vi "Main.vi"(11 "Module Admin":refnum<class "Delacor_lib_QMH_Cloneable Module Admin.lvclass">) -> ()   [LabVIEW 2022 SP3, in "Serial-Com-Module.lvlib"]
doc: "This template is based off of the Queued Message Handler design pattern and the Queued Message Handler project template that ships with LabVIEW.\n\nThe main difference is that the queue is private to this module and communication between modules is performed via Broadcast and Request events.\n\nRequest events are wrapped in public API methods and are handled in the Event Handling Loop (EHL) of this VI. Any module can register for Broadcast events sent by this module. The EHL generates messages based on user interface actions.\n\nThe Message Handling Loop (MHL) processes messages generated by the EHL, or by other messages. The messages are string values, so new messages can be added easily to the Message Cases case structure in the MHL. Each message cluster can also provide an optional value for Message Data, which is a variant that can be converted to whatever message-specific data is required.\n_____\nBased on DQMH Project Template 6.1.0.94."
uses:
  Serial-Com-Module.lvlib
  <vilib>/Delacor/Delacor QMH/Libraries/Message Queue_class/Delacor_lib_QMH_Message Queue.lvclass
  Module Data--cluster.ctl
  <vilib>/Utility/miscctls.llb/LVPointTypeDef.ctl
  <vilib>/Utility/error.llb/Error Cluster From Error Code.vi
  <vilib>/ErrorRing/Error Ring.xnode
  <vilib>/Delacor/Delacor QMH/Libraries/Message Queue_class/Delacor_lib_QMH_Enqueue Message (Single).vi
  Stop Argument--cluster.ctl
  <vilib>/Delacor/Delacor QMH/Libraries/Cloneable Module Admin_class/Delacor_lib_QMH_Cloneable Module Admin.lvclass
  Dependencies/Serial-Com-Library.lvlibp/Serial Base Class/Serial Base.lvclass
  Init Serial (Reply Payload)--cluster.ctl
  Dependencies/Serial-Com-Library.lvlibp/Serial Base Class/Object Argument--cluster.ctl
  Init Serial Argument--cluster.ctl
  Open Port (Reply Payload)--cluster.ctl
  Open Port Argument--cluster.ctl
  Close Port (Reply Payload)--cluster.ctl
  Close Port Argument--cluster.ctl
  Read Buffer (Reply Payload)--cluster.ctl
  Read Buffer Argument--cluster.ctl
  Send (Reply Payload)--cluster.ctl
  Send Argument--cluster.ctl
  Send Line (Reply Payload)--cluster.ctl
  Dependencies/Serial-Com-Library.lvlibp/Serial Base Class/Termination Character--enum.ctl
  Send Line Argument--cluster.ctl
panel:
  out "error out":errorcluster
  out "Status":string
  in  "Simulate EHL Error":bool
  in  "Simulate MHL Error":bool
  # "Other QMH Modules communicate with this Module via its Public API (wrappers for its Request Events).\n\nThis Module communicates with other Modules via its Broadcast Events.\nAny module that wants to get these messages, just registers for this module's Broadcast events."
  # "This template is for the Delacor Modified Queued Message Handler design pattern.\n\nSee the block diagram for more information on how to use this template."
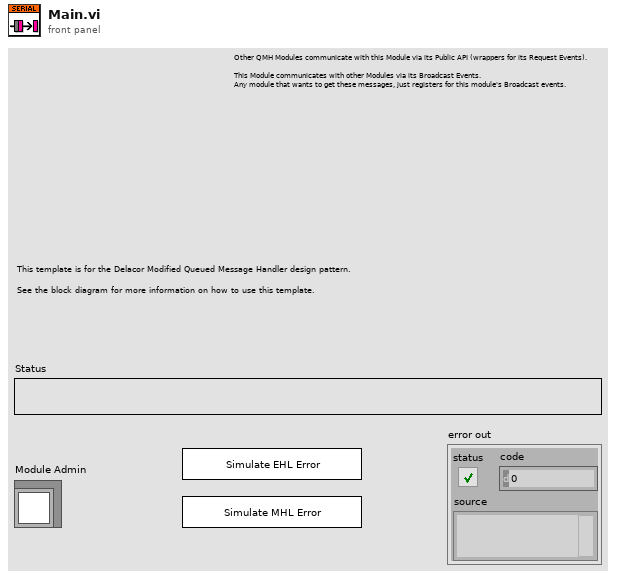
[diagram p1: front panel]
types:
  T1 = typedef "Serial-Com-Module.lvlib/Request Events--cluster.ctl" = cluster{"Stop Module":refnum<user-event>, "Show Panel":refnum<user-event>, "Hide Panel":refnum<user-event>, "Show Diagram":refnum<user-event>, "Get Module Execution Status":refnum<user-event>, "Init Serial":refnum<user-event>, "Open Port":refnum<user-event>, "Close Port":refnum<user-event>, "Read Buffer":refnum<user-event>, "Send":refnum<user-event>, "Send Line":refnum<user-event>}
  T2 = typedef "Serial-Com-Module.lvlib/Module Data--cluster.ctl" = cluster{"Status":string, "Serial Com Obj":refnum<class "Serial Base.lvclass">}
  T3 = enum32{"invalid lock state", "Not Locked", "Locked (No Password)", "Password-protected"}
  T4 = typedef "Serial-Com-Module.lvlib/Stop Argument--cluster.ctl" = cluster{"Module ID":i32, "Origin":string, "Exit via Stop Module Req?":bool, "Wait for Module to stop?":bool}
  T5 = typedef "Serial-Com-Module.lvlib/Init Serial Argument--cluster.ctl" = cluster{"Module ID":i32, "Serial Config":T6, "Wait Notifier":refnum<notifier>, "wait for reply":bool}
  T6 = typedef "Serial-Com-Library.lvlibp/Serial Base.lvclass/Object Argument--cluster.ctl" = cluster{"Com Port":refnum<visa-resource-name>, "baud rate":u32, "data bits":u16, "parity":enum16{"None", "Odd", "Even", "Mark", "Space"}, "timeout ":u32}
  T7 = typedef "Serial-Com-Module.lvlib/Open Port Argument--cluster.ctl" = cluster{"Module ID":i32, "Open Port?":bool, "Wait Notifier":refnum<notifier>, "wait for reply":bool}
  T8 = typedef "Serial-Com-Module.lvlib/Close Port Argument--cluster.ctl" = cluster{"Module ID":i32, "ClosePort?":bool, "Wait Notifier":refnum<notifier>, "wait for reply":bool}
  T9 = typedef "Serial-Com-Module.lvlib/Read Buffer Argument--cluster.ctl" = cluster{"Module ID":i32, "pre-read delay":i16, "Wait Notifier":refnum<notifier>, "wait for reply":bool}
  T10 = typedef "Serial-Com-Module.lvlib/Send Argument--cluster.ctl" = cluster{"Module ID":i32, "data":string, "Wait Notifier":refnum<notifier>, "wait for reply":bool}
  T11 = typedef "Serial-Com-Module.lvlib/Send Line Argument--cluster.ctl" = cluster{"Module ID":i32, "Termination Char":T12, "data":string, "Wait Notifier":refnum<notifier>, "wait for reply":bool}
  T12 = typedef "Serial-Com-Library.lvlibp/Serial Base.lvclass/Termination Character--enum.ctl" = enum16{"none", "\\r\\n", "\\r", "\\n"}
  T13 = typedef "LVPointTypeDef.ctl" = cluster{"Horizontal":i16, "Vertical":i16}
  T14 = enum32{"Invalid", "Standard", "Closed", "Hidden", "Minimized", "Maximized"}
  T15 = typedef "Serial-Com-Module.lvlib/Init Serial (Reply Payload)--cluster.ctl" = cluster{"error":errorcluster}
  T16 = typedef "Serial-Com-Module.lvlib/Open Port (Reply Payload)--cluster.ctl" = cluster{"error":errorcluster}
  T17 = typedef "Serial-Com-Module.lvlib/Close Port (Reply Payload)--cluster.ctl" = cluster{"error":errorcluster}
  T18 = typedef "Serial-Com-Module.lvlib/Read Buffer (Reply Payload)--cluster.ctl" = cluster{"buffer output":string, "bytes count":i16, "error":errorcluster}
  T19 = typedef "Serial-Com-Module.lvlib/Send (Reply Payload)--cluster.ctl" = cluster{"bytes count sent":u32, "error":errorcluster}
  T20 = typedef "Serial-Com-Module.lvlib/Send Line (Reply Payload)--cluster.ctl" = cluster{"bytes count":u32, "error":errorcluster}
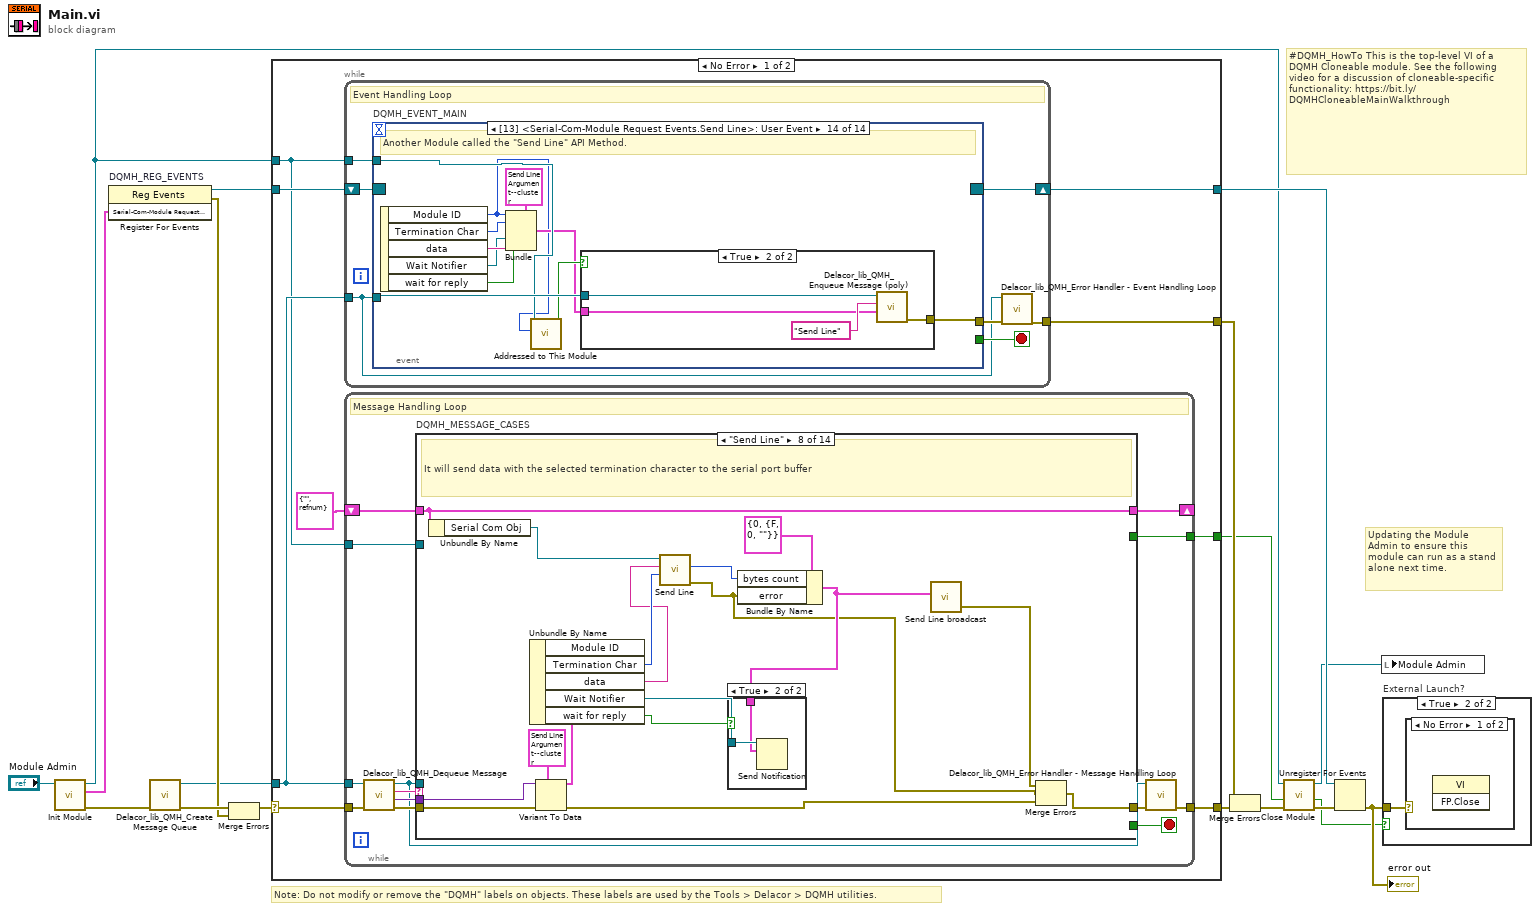
[diagram p0: block diagram]
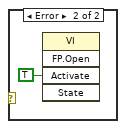
[diagram p3: hidden frame]
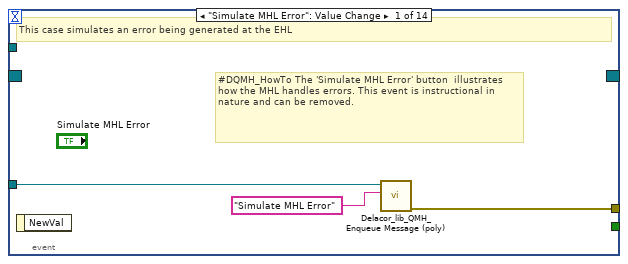
[diagram p4: hidden frame]
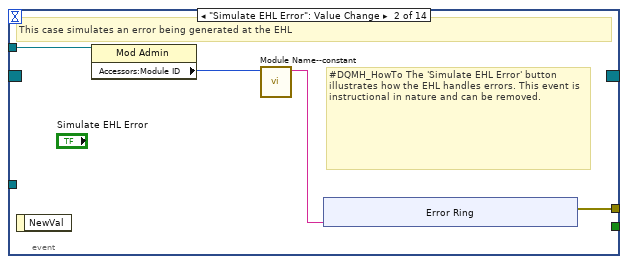
[diagram p5: hidden frame]
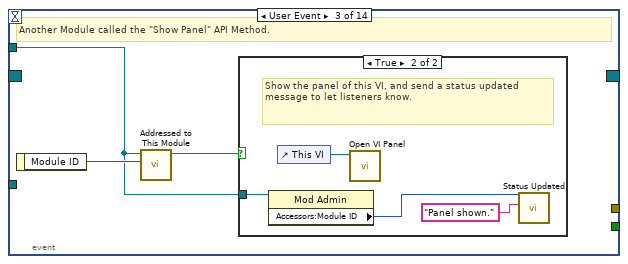
[diagram p6: hidden frame]
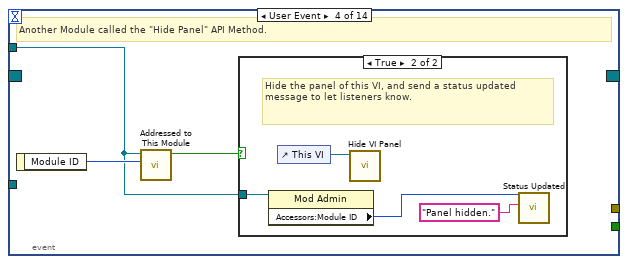
[diagram p8: hidden frame]
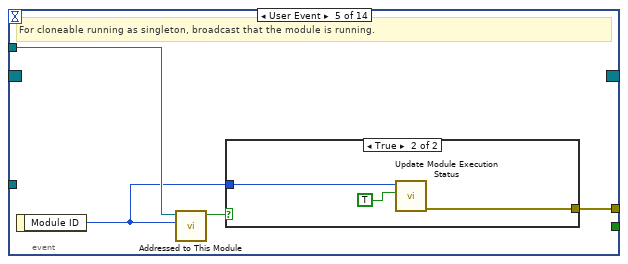
[diagram p10: hidden frame]
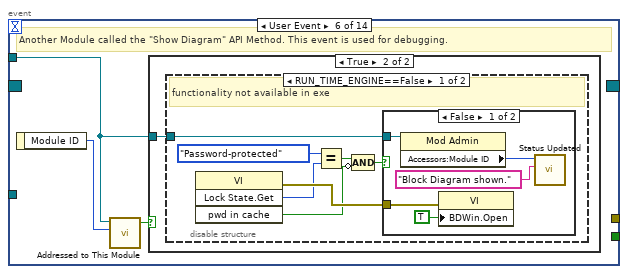
[diagram p12: hidden frame]
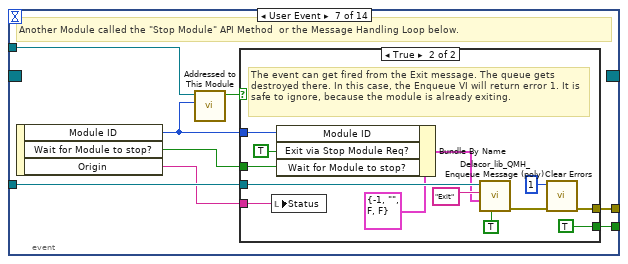
[diagram p16: hidden frame]
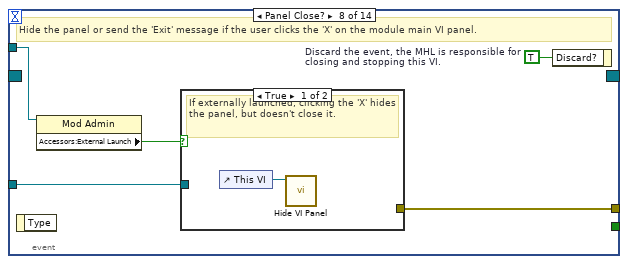
[diagram p18: hidden frame]
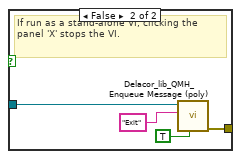
[diagram p19: hidden frame]
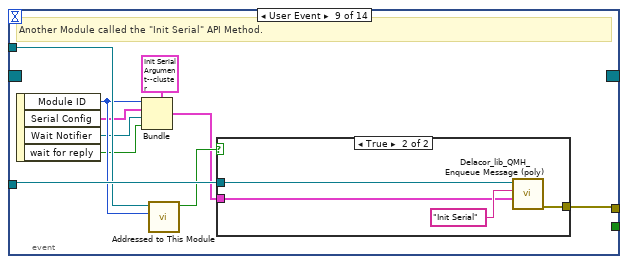
[diagram p20: hidden frame]
diagram:
  # "#DQMH_HowTo This is the top-level VI of a DQMH Cloneable module. See the following video for a discussion of cloneable-specific functionality: https://bit.ly/DQMHCloneableMainWalkthrough"
  # "Note: Do not modify or remove the \"DQMH\" labels on objects. These labels are used by the Tools > Delacor > DQMH utilities."
  # "Updating the Module Admin to ensure this module can run as a stand alone next time."
  n1 = call "Init Module.vi"("Cloneable Module Admin in"="Module Admin") -> ("error out"=w15:errorcluster, "Serial-Com-Module Request Events"=w7:T1, "Cloneable Module Admin out"=w4:refnum<class "Delacor_lib_QMH_Cloneable Module Admin.lvclass">)  [unwired: 8 in]
  n2 = register-events "DQMH_REG_EVENTS"(w7) -> (reference out=w8:refnum<event-registration>, error out=w10:errorcluster)  [unwired: 2 in]
  n3 = call <vilib>:"Delacor_lib_QMH_Create Message Queue.vi"("error in"=w15) -> ("error out"=w12:errorcluster, "Message Queue"=w6:refnum<class "Delacor_lib_QMH_Message Queue.lvclass">)  [unwired: 9 in]
  n4 = Merge Errors(w12, w10) -> (w11:errorcluster)
  n5 = case shown="No Error" w11 {
    selector: w11 -> [w25 w428]
    tunnel: [w27 w427] -> w16
    tunnel: [w24 w435] -> w9
    tunnel: w8 -> [w22 w435]
    tunnel: w6 -> [w21 w426]
    tunnel: [w26 _] -> w17
    tunnel: w4 -> [w20 w431]
    tunnel: [w19 _] -> w2
    frame No Error {
      n6 = while {
        tunnel: w21 -> [w28]
        shift-right: [w31] -> w24
        shift-left: w22 -> [w32]
        tunnel: [w33] -> w26
        tunnel: w20 -> [w29]
        stop <- w30 stop-if-true
        # "Event Handling Loop"
        n7 = event "DQMH_EVENT_MAIN" shown="[13] <Serial-Com-Module Request Events.Send Line>: User Event" {
          selector: w32 -> [_ _ _ _ _ _ _ _ _ _ _ _ _ _]
          dyn-events: [_ _ _ _ _ _ _ _ _ _ _ _ _ _] -> w31
          timeout: _ -> [_ _ _ _ _ _ _ _ _ _ _ _ _ _]
          tunnel: [_ _ _ _ _ _ w89 _ _ _ _ _ _ _] -> w30
          tunnel: w28 -> [w36 _ _ _ _ _ w92 w108 w126 w140 w154 w168 w182 w197]
          tunnel: [w37 w41 _ _ w66 _ w93 w111 w117 w131 w145 w159 w173 w187] -> w34
          tunnel: w29 -> [_ w40 w49 w56 w64 w70 w91 w109 w124 w138 w152 w166 w180 w195]
          event "Simulate MHL Error": Value Change {
            # "#DQMH_HowTo The 'Simulate MHL Error' button  illustrates how the MHL handles errors. This event is instructional in nature and can be removed."
            # "This case simulates an error being generated at the EHL"
            n8 = event-data() -> ()  [unwired: 1 in, 1 out]
            n9 = call-poly <vilib>:"Delacor_lib_QMH_Enqueue Message (poly).vi"("Message"="Simulate MHL Error", "Message Queue in"=w36) -> ("error out"=w37:errorcluster)  [unwired: 8 in, 1 out]
          }
          event "Simulate EHL Error": Value Change {
            # "#DQMH_HowTo The 'Simulate EHL Error' button  illustrates how the EHL handles errors. This event is instructional in nature and can be removed."
            # "This case simulates an error being generated at the EHL"
            n10 = event-data() -> ()  [unwired: 1 in, 1 out]
            n11 = property class="Mod Admin"(reference=w40) -> ("Accessors:Module ID"=w39:i32)  [unwired: 1 in, 2 out]
            n12 = call "Module Name--constant.vi"("Module ID"=w39) -> ("Module Name"=w38:string)  [unwired: 10 in]
            n13 = xnode "Error Ring"("parameter 0"=w38) -> ("error out"=w41:errorcluster)
          }
          event User Event {
            # "Another Module called the \"Show Panel\" API Method."
            n14 = event-data() -> ("Module ID"=w50:i32)  [unwired: 1 in]
            n15 = call "Addressed to This Module.vi"("Module ID from Argument"=w50, "Module Admin"=w49) -> ("Addressed to this instance?"=w51:bool)  [unwired: 8 in, 1 out]
            n16 = case shown="True" w51 {
              tunnel: w49 -> [_ w53]
              frame False {
              }
              frame True {
                # "Show the panel of this VI, and send a status updated message to let listeners know."
                n17 = property class="Mod Admin"(reference=w53) -> ("Accessors:Module ID"=w52:i32)  [unwired: 1 in, 2 out]
                n18 = control-ref of="This VI"() -> (w55:refnum<vi>)
                n19 = call "Open VI Panel.vi"("VI"=w55) -> ()  [unwired: 10 in, 1 out]
                n20 = call "Status Updated.vi"("Status"="Panel shown." ("format string"), "Module ID"=w52) -> ()  [unwired: 9 in, 1 out]
              }
            }
          }
          event User Event {
            # "Another Module called the \"Hide Panel\" API Method."
            n21 = event-data() -> ("Module ID"=w57:i32)  [unwired: 1 in]
            n22 = call "Addressed to This Module.vi"("Module ID from Argument"=w57, "Module Admin"=w56) -> ("Addressed to this instance?"=w58:bool)  [unwired: 8 in, 1 out]
            n23 = case shown="True" w58 {
              tunnel: w56 -> [_ w60]
              frame False {
              }
              frame True {
                # "Hide the panel of this VI, and send a status updated message to let listeners know."
                n24 = property class="Mod Admin"(reference=w60) -> ("Accessors:Module ID"=w59:i32)  [unwired: 1 in, 2 out]
                n25 = control-ref of="This VI"() -> (w62:refnum<vi>)
                n26 = call "Hide VI Panel.vi"("VI"=w62) -> ()  [unwired: 10 in, 1 out]
                n27 = call "Status Updated.vi"("Status"="Panel hidden." ("format string"), "Module ID"=w59) -> ()  [unwired: 9 in, 1 out]
              }
            }
          }
          event User Event {
            # "For cloneable running as singleton, broadcast that the module is running."
            n28 = event-data() -> ("Module ID"=w63:i32)  [unwired: 1 in]
            n29 = call "Addressed to This Module.vi"("Module ID from Argument"=w63, "Module Admin"=w64) -> ("Addressed to this instance?"=w65:bool)  [unwired: 8 in, 1 out]
            n30 = case shown="True" w65 {
              tunnel: [_ w69] -> w66
              tunnel: w63 -> [_ w68]
              frame False {
              }
              frame True {
                n31 = call "Update Module Execution Status.vi"("Running?"=TRUE, "Module ID"=w68) -> ("error out"=w69:errorcluster)  [unwired: 9 in]
              }
            }
          }
          event User Event {
            # "Another Module called the \"Show Diagram\" API Method. This event is used for debugging."
            n32 = event-data() -> ("Module ID"=w71:i32)  [unwired: 1 in]
            n33 = call "Addressed to This Module.vi"("Module ID from Argument"=w71, "Module Admin"=w70) -> ("Addressed to this instance?"=w72:bool)  [unwired: 8 in, 1 out]
            n34 = case shown="True" w72 {
              tunnel: w70 -> [_ w73]
              frame False {
              }
              frame True {
                n35 = disable-structure shown="RUN_TIME_ENGINE==False" {
                  disable-tunnel: w73 -> [w74 _]
                  frame condition #0 (active) {
                    # "functionality not available in exe"
                    n36 = invoke class="VI" method="Lock State.Get"() -> (error out=w80:errorcluster, "Get Lock State"=w79:T3, "pwd in cache"=w76:bool)  [unwired: 4 in, 1 out]
                    n37 = Equal?(x=T3."Password-protected", y=w79) -> (x = y?=w77:bool)
                    n38 = Compound Arithmetic op=AND(w77, invert w76) -> (w75:bool)
                    n39 = case shown="False" w75 {
                      tunnel: w80 -> [w85 _]
                      tunnel: w74 -> [w82 _]
                      frame False {
                        n40 = property class="Mod Admin"(reference=w82) -> ("Accessors:Module ID"=w81:i32)  [unwired: 1 in, 2 out]
                        n41 = property class="VI"(error in=w85, "BDWin.Open"=TRUE ("Block Diagram Window:Open")) -> ()  [unwired: 1 in, 2 out]
                        n42 = call "Status Updated.vi"("Status"="Block Diagram shown." ("format string"), "Module ID"=w81) -> ()  [unwired: 9 in, 1 out]
                      }
                      frame True {
                        # "Password-protected VI, and the password is not in the cache. Do not show the diagram."
                      }
                    }
                  }
                  frame condition #1 {
                  }
                }
              }
            }
          }
          event User Event {
            # "Another Module called the \"Stop Module\" API Method  or the Message Handling Loop below."
            n43 = event-data() -> ("Module ID"=w87:i32, "Wait for Module to stop?"=w88:bool, "Origin"=w86:string)  [unwired: 1 in]
            n44 = call "Addressed to This Module.vi"("Module ID from Argument"=w87, "Module Admin"=w91) -> ("Addressed to this instance?"=w90:bool)  [unwired: 8 in, 1 out]
            n45 = case shown="True" w90 {
              tunnel: [_ w105] -> w93
              tunnel: w92 -> [_ w101]
              tunnel: [_ TRUE] -> w89
              tunnel: w88 -> [_ w96]
              tunnel: w87 -> [_ w98]
              tunnel: w86 -> [_ w94]
              frame False {
              }
              frame True {
                # "The event can get fired from the Exit message. The queue gets destroyed there. In this case, the Enqueue VI will return error 1. It is safe to ignore, because the module is already exiting."
                n46 = local write "Status"(w94) -> ()
                n47 = Bundle By Name(cluster=T4 {"Module ID"=-1, "Origin"="", "Exit via Stop Module Req?"=FALSE, "Wait for Module to stop?"=FALSE} ("Stop Argument"), "Module ID"=w98, "Exit via Stop Module Req?"=TRUE, "Wait for Module to stop?"=w96) -> (w95:T4)
                n48 = call-poly <vilib>:"Delacor_lib_QMH_Enqueue Message (poly).vi"("Priority Message? (F)"=TRUE, "Message Data"=w95, "Message"="Exit", "Message Queue in"=w101) -> ("error out"=w106:errorcluster)  [unwired: 6 in, 1 out]
                n49 = call <vilib>:"Clear Errors.vi"("error in (no error)"=w106, "specific error code to clear (0: all)"=1) -> ("error out"=w105:errorcluster)  [unwired: 4 in, 1 out]
              }
            }
          }
          event Panel Close? {
            w110 = TRUE  # Discard the event, the MHL is responsible for closing and stopping this VI.
            # "Hide the panel or send the 'Exit' message if the user clicks the 'X' on the module main VI panel."
            n50 = event-data() -> ()  [unwired: 1 in, 1 out]
            n51 = property class="Mod Admin"(reference=w109) -> ("Accessors:External Launch"=w107:bool)  [unwired: 1 in, 2 out]
            n52 = case shown="True" w107 {
              tunnel: w108 -> [_ w115]
              tunnel: [_ w116] -> w111
              frame True {
                # "If externally launched, clicking the 'X' hides the panel, but doesn't close it."
                n53 = control-ref of="This VI"() -> (w112:refnum<vi>)
                n54 = call "Hide VI Panel.vi"("VI"=w112) -> ()  [unwired: 10 in, 1 out]
              }
              frame False {
                # "If run as a stand-alone VI, clicking the panel 'X' stops the VI."
                n55 = call-poly <vilib>:"Delacor_lib_QMH_Enqueue Message (poly).vi"("Priority Message? (F)"=TRUE, "Message"="Exit", "Message Queue in"=w115) -> ("error out"=w116:errorcluster)  [unwired: 7 in, 1 out]
              }
            }
            n56 = event-data("Discard?"=w110) -> ()  [unwired: 1 in, 1 out]
          }
          event User Event {
            # "Another Module called the \"Init Serial\" API Method."
            n57 = event-data() -> ("Module ID"=w121:i32, "Serial Config"=w120:T6, "Wait Notifier"=w119:refnum<notifier>, "wait for reply"=w118:bool)  [unwired: 1 in]
            n58 = Bundle(cluster=T5 {"Module ID"=-1, "Serial Config"={"Com Port"="", "baud rate"=0, "data bits"=8, "parity"=enum."None", "timeout "=10000}, "Wait Notifier"=refnum, "wait for reply"=FALSE} ("Init Serial Argument"), "Module ID"=w121, "Serial Config"=w120, "Wait Notifier"=w119, "wait for reply"=w118) -> (w122:T5)
            n59 = call "Addressed to This Module.vi"("Module ID from Argument"=w121, "Module Admin"=w124) -> ("Addressed to this instance?"=w125:bool)  [unwired: 8 in, 1 out]
            n60 = case shown="True" w125 {
              tunnel: w126 -> [_ w130]
              tunnel: w122 -> [_ w128]
              tunnel: [_ w127] -> w117
              frame False {
              }
              frame True {
                n61 = call-poly <vilib>:"Delacor_lib_QMH_Enqueue Message (poly).vi"("Message Data"=w128, "Message"="Init Serial", "Message Queue in"=w130) -> ("error out"=w127:errorcluster)  [unwired: 7 in, 1 out]
              }
            }
          }
          event User Event {
            # "Another Module called the \"Open Port\" API Method."
            n62 = event-data() -> ("Module ID"=w135:i32, "Open Port?"=w134:bool, "Wait Notifier"=w133:refnum<notifier>, "wait for reply"=w132:bool)  [unwired: 1 in]
            n63 = Bundle(cluster=T7 {"Module ID"=-1, "Open Port?"=FALSE, "Wait Notifier"=refnum, "wait for reply"=FALSE} ("Open Port Argument"), "Module ID"=w135, "Open Port?"=w134, "Wait Notifier"=w133, "wait for reply"=w132) -> (w136:T7)
            n64 = call "Addressed to This Module.vi"("Module ID from Argument"=w135, "Module Admin"=w138) -> ("Addressed to this instance?"=w139:bool)  [unwired: 8 in, 1 out]
            n65 = case shown="True" w139 {
              tunnel: w140 -> [_ w144]
              tunnel: w136 -> [_ w142]
              tunnel: [_ w141] -> w131
              frame False {
              }
              frame True {
                n66 = call-poly <vilib>:"Delacor_lib_QMH_Enqueue Message (poly).vi"("Message Data"=w142, "Message"="Open Port", "Message Queue in"=w144) -> ("error out"=w141:errorcluster)  [unwired: 7 in, 1 out]
              }
            }
          }
          event User Event {
            # "Another Module called the \"Close Port\" API Method."
            n67 = event-data() -> ("Module ID"=w149:i32, "ClosePort?"=w148:bool, "Wait Notifier"=w147:refnum<notifier>, "wait for reply"=w146:bool)  [unwired: 1 in]
            n68 = Bundle(cluster=T8 {"Module ID"=-1, "ClosePort?"=FALSE, "Wait Notifier"=refnum, "wait for reply"=FALSE} ("Close Port Argument"), "Module ID"=w149, "ClosePort?"=w148, "Wait Notifier"=w147, "wait for reply"=w146) -> (w150:T8)
            n69 = call "Addressed to This Module.vi"("Module ID from Argument"=w149, "Module Admin"=w152) -> ("Addressed to this instance?"=w153:bool)  [unwired: 8 in, 1 out]
            n70 = case shown="True" w153 {
              tunnel: w154 -> [_ w158]
              tunnel: w150 -> [_ w156]
              tunnel: [_ w155] -> w145
              frame False {
              }
              frame True {
                n71 = call-poly <vilib>:"Delacor_lib_QMH_Enqueue Message (poly).vi"("Message Data"=w156, "Message"="Close Port", "Message Queue in"=w158) -> ("error out"=w155:errorcluster)  [unwired: 7 in, 1 out]
              }
            }
          }
          event User Event {
            # "Another Module called the \"Read Buffer\" API Method."
            n72 = event-data() -> ("Module ID"=w163:i32, "pre-read delay"=w162:i16, "Wait Notifier"=w161:refnum<notifier>, "wait for reply"=w160:bool)  [unwired: 1 in]
            n73 = Bundle(cluster=T9 {"Module ID"=-1, "pre-read delay"=-1, "Wait Notifier"=refnum, "wait for reply"=FALSE} ("Read Buffer Argument"), "Module ID"=w163, "pre-read delay"=w162, "Wait Notifier"=w161, "wait for reply"=w160) -> (w164:T9)
            n74 = call "Addressed to This Module.vi"("Module ID from Argument"=w163, "Module Admin"=w166) -> ("Addressed to this instance?"=w167:bool)  [unwired: 8 in, 1 out]
            n75 = case shown="True" w167 {
              tunnel: w168 -> [_ w172]
              tunnel: w164 -> [_ w170]
              tunnel: [_ w169] -> w159
              frame False {
              }
              frame True {
                n76 = call-poly <vilib>:"Delacor_lib_QMH_Enqueue Message (poly).vi"("Message Data"=w170, "Message"="Read Buffer", "Message Queue in"=w172) -> ("error out"=w169:errorcluster)  [unwired: 7 in, 1 out]
              }
            }
          }
          event User Event {
            # "Another Module called the \"Send\" API Method."
            n77 = event-data() -> ("Module ID"=w177:i32, "data"=w176:string, "Wait Notifier"=w175:refnum<notifier>, "wait for reply"=w174:bool)  [unwired: 1 in]
            n78 = Bundle(cluster=T10 {"Module ID"=-1, "data"="", "Wait Notifier"=refnum, "wait for reply"=FALSE} ("Send Argument"), "Module ID"=w177, "data"=w176, "Wait Notifier"=w175, "wait for reply"=w174) -> (w178:T10)
            n79 = call "Addressed to This Module.vi"("Module ID from Argument"=w177, "Module Admin"=w180) -> ("Addressed to this instance?"=w181:bool)  [unwired: 8 in, 1 out]
            n80 = case shown="True" w181 {
              tunnel: w182 -> [_ w186]
              tunnel: w178 -> [_ w184]
              tunnel: [_ w183] -> w173
              frame False {
              }
              frame True {
                n81 = call-poly <vilib>:"Delacor_lib_QMH_Enqueue Message (poly).vi"("Message Data"=w184, "Message"="Send", "Message Queue in"=w186) -> ("error out"=w183:errorcluster)  [unwired: 7 in, 1 out]
              }
            }
          }
          event User Event {
            # "Another Module called the \"Send Line\" API Method."
            n82 = event-data() -> ("Module ID"=w192:i32, "Termination Char"=w191:T12, "data"=w190:string, "Wait Notifier"=w189:refnum<notifier>, "wait for reply"=w188:bool)  [unwired: 1 in]
            n83 = Bundle(cluster=T11 {"Module ID"=-1, "Termination Char"=enum."none", "data"="", "Wait Notifier"=refnum, "wait for reply"=FALSE} ("Send Line Argument"), "Module ID"=w192, "Termination Char"=w191, "data"=w190, "Wait Notifier"=w189, "wait for reply"=w188) -> (w193:T11)
            n84 = call "Addressed to This Module.vi"("Module ID from Argument"=w192, "Module Admin"=w195) -> ("Addressed to this instance?"=w196:bool)  [unwired: 8 in, 1 out]
            n85 = case shown="True" w196 {
              tunnel: w197 -> [_ w201]
              tunnel: w193 -> [_ w199]
              tunnel: [_ w198] -> w187
              frame False {
              }
              frame True {
                n86 = call-poly <vilib>:"Delacor_lib_QMH_Enqueue Message (poly).vi"("Message Data"=w199, "Message"="Send Line", "Message Queue in"=w201) -> ("error out"=w198:errorcluster)  [unwired: 7 in, 1 out]
              }
            }
          }
        }
        n87 = call-dynamic "Delacor_lib_QMH_Error Handler - Event Handling Loop.vi"("error in"=w34, "Message Queue in"=w28) -> ("dup error in"=w33:errorcluster)  [unwired: 8 in, 1 out]
      }
      n88 = while {
        tunnel: w21 -> [w205]
        shift-right: [w209] -> _
        shift-left: T2 {"Status"="", "Serial Com Obj"=refnum} ("Data Cluster") -> [w210]
        tunnel: w25 -> [w213]
        tunnel: [w211] -> w27
        tunnel: w20 -> [w203]
        tunnel: [w202] -> w19
        stop <- w208 stop-if-true
        # "Message Handling Loop"
        n89 = call-dynamic "Delacor_lib_QMH_Dequeue Message.vi"("error in"=w213, "Message Queue in"=w205) -> ("error out"=w212:errorcluster, "Message Data"=w206:variant, "Message"=w207:string, "Message Queue out"=w204:refnum<class "Delacor_lib_QMH_Message Queue.lvclass">)  [unwired: 6 in]
        n90 = case "DQMH_MESSAGE_CASES" shown="\"Send Line\"" w207 {
          selector: w207 -> [_ _ _ _ _ _ _ _ _ _ _ _ _ w413]
          tunnel: w204 -> [_ _ _ _ _ _ _ _ _ _ w364 _ w403 _]
          tunnel: w212 -> [w233 w237 w250 w277 w295 w316 w336 w355 w360 w362 w373 w386 w409 w415]
          tunnel: [w231 w237 w244 w270 w286 w307 w327 w346 w359 w362 w369 w385 w406 w416] -> w214
          tunnel: w210 -> [w224 w236 w243 w268 w284 w302 w323 w345 w358 w361 w368 w383 w402 w414]
          tunnel: [w223 w236 w242 w267 w282 w300 w322 w345 w358 w361 w368 w383 w402 w414] -> w209
          tunnel: [_ _ _ _ _ _ _ _ _ _ _ _ w401 _] -> w208
          tunnel: w206 -> [_ _ w249 w275 w293 w314 w334 w353 _ _ w367 _ w399 _]
          tunnel: w203 -> [w218 _ _ _ _ _ _ _ _ _ w366 w381 w395 w411]
          tunnel: [_ _ _ _ _ _ _ _ _ _ _ _ w397 _] -> w202
          frame "Initialize" {
            w215 = "Initial Message" ("Initial Message")
            # "#CodeNeeded - Initialize the appearance of the front panel."
            # "#CodeNeeded - Initialize your state data here."
            # "Initialize - Any operation that needs to be done before the module can receive messages. Synchronize Caller Events.vi will inform Start Module.vi that the module has launched and is ready to receive messages. Module Did Init.vi will broadcast that the module initialized."
            n91 = call "Synchronize Caller Events.vi"("error in (no error)"=w233, "Module Admin"=w218) -> ("error out"=w232:errorcluster, "Module Admin out"=w217:refnum<class "Delacor_lib_QMH_Cloneable Module Admin.lvclass">)  [unwired: 8 in]
            n92 = property class="Mod Admin"(reference=w217) -> ("Accessors:Module ID"=w220:i32, "Accessors:External Launch"=w219:bool)  [unwired: 1 in, 2 out]
            n93 = call "Module Name--constant.vi"("Module ID"=w220) -> ("Module Name"=w228:string)  [unwired: 10 in]
            n94 = property class="VI"("Front Panel.Title"=w228) -> (reference out=w230:refnum<vi>, error out=w235:errorcluster)  [unwired: 2 in]
            n95 = Select(t=T14."Hidden" ("State"), s=w219, f=T14."Standard" ("State")) -> (s? t:f=w225:T14)
            n96 = invoke class="VI" method="FP.Open"(reference=w230, error in=w235, "State"=w225) -> (reference out=w229:refnum<vi>, error out=w234:errorcluster)  [unwired: 2 in, 3 out]
            n97 = call "Module Name--constant.vi"("Module ID"=w220) -> ("Module Name"=w221:string)  [unwired: 10 in]
            n98 = Bundle By Name(cluster=w224, "Status"=w215) -> (w223:T2)
            n99 = invoke class="VI" method="FP.Center"(reference=w229, error in=w234) -> ()  [unwired: 1 in, 3 out]
            n100 = property on="Pane" class="Pane"("Origin"=T13 {"Horizontal"=0, "Vertical"=0}) -> ()  [unwired: 2 in, 2 out]
            n101 = call "Module Did Init.vi"("error in (no error)"=w232, "Initialized?"=TRUE, "Origin"=w221, "Module ID"=w220) -> ("error out"=w231:errorcluster)  [unwired: 7 in]
            "Status" <- w215
          }
          frame "---Module Specific---" {
            # "Separator -- The following cases handle messages specific to this Module."
          }
          frame "Init Serial" {
            # "It will populate the config parameters required before open the serial port"
            n102 = Variant To Data(error in=w250, type=T5 {"Module ID"=-1, "Serial Config"={"Com Port"="", "baud rate"=0, "data bits"=8, "parity"=enum."None", "timeout "=10000}, "Wait Notifier"=refnum, "wait for reply"=FALSE} ("Init Serial Argument"), Variant=w249) -> (data=w247:T5, error out=w241:errorcluster)
            n103 = Unbundle By Name(w247) -> ("Serial Config"=w239:T6, "Wait Notifier"=w246:refnum<notifier>, "wait for reply"=w245:bool)  [unwired: 1 out]
            n104 = case shown="True" w245 {
              tunnel: w246 -> [_ w261]
              tunnel: w239 -> [_ w258]
              tunnel: [errorcluster {"status"=FALSE, "code"=0, "source"=""} ("error out") w256] -> w240
              tunnel: [refnum<class "Serial Base.lvclass"> refnum ("Serial-Com-Library.lvlibp:Serial Base.lvclass") w255] -> w238
              frame False {
              }
              frame True {
                n105 = call-dynamic "Init.vi"("error in (no error)"=errorcluster {"status"=FALSE, "code"=0, "source"=""}, "Serial Config"=w258, "Serial Base in"=refnum<class "Serial Base.lvclass"> refnum ("Serial-Com-Library.lvlibp:Serial Base.lvclass")) -> ("error out"=w254:errorcluster, "Serial Base out"=w255:refnum<class "Serial Base.lvclass">)  [unwired: 7 in]
                n106 = Bundle By Name(cluster=T15 {"error"={"status"=FALSE, "code"=0, "source"=""}} ("Init Serial (Reply Payload)"), "error"=w254) -> (w259:T15)
                n107 = call "Serial Did Init.vi"("error in"=w254, "Reply Payload"=w259) -> ("error out"=w256:errorcluster)  [unwired: 9 in]
                n108 = Send Notification(notification=w259, notifier=w261) -> ()  [unwired: 1 in, 2 out]
              }
            }
            n109 = Bundle By Name(cluster=w243, "Serial Com Obj"=w238) -> (w242:T2)
            n110 = Merge Errors(w240, w241) -> (w244:errorcluster)
          }
          frame "Open Port" {
            # "It will open the serial port with the config previous set in the init event."
            n111 = Unbundle By Name(w268) -> ("Serial Com Obj"=w269:refnum<class "Serial Base.lvclass">)
            n112 = Variant To Data(error in=w277, type=T7 {"Module ID"=-1, "Open Port?"=FALSE, "Wait Notifier"=refnum, "wait for reply"=FALSE} ("Open Port Argument"), Variant=w275) -> (data=w273:T7, error out=w276:errorcluster)
            n113 = Unbundle By Name(w273) -> ("Wait Notifier"=w272:refnum<notifier>, "wait for reply"=w271:bool)  [unwired: 2 out]
            n114 = call-dynamic "Open port.vi"("Serial Base in"=w269) -> ("error out"=w266:errorcluster, "Serial Base out"=w265:refnum<class "Serial Base.lvclass">)  [unwired: 9 in]
            n115 = Bundle By Name(cluster=T16 {"error"={"status"=FALSE, "code"=0, "source"=""}} ("Open Port (Reply Payload)"), "error"=w266) -> (w264:T16)
            n116 = case shown="True" w271 {
              tunnel: w272 -> [_ w279]
              tunnel: w264 -> [_ w278]
              frame False {
              }
              frame True {
                n117 = Send Notification(notification=w278, notifier=w279) -> ()  [unwired: 1 in, 2 out]
              }
            }
            n118 = call "Serial Port Did Open.vi"("error in"=w266, "Reply Payload"=w264) -> ("error out"=w263:errorcluster)  [unwired: 9 in]
            n119 = Bundle By Name(cluster=w268, "Serial Com Obj"=w265) -> (w267:T2)
            n120 = Merge Errors(w263, w276) -> (w270:errorcluster)
          }
          frame "Close Port" {
            # "It will close the serial port"
            n121 = Unbundle By Name(w284) -> ("Serial Com Obj"=w285:refnum<class "Serial Base.lvclass">)
            n122 = Variant To Data(error in=w295, type=T8 {"Module ID"=-1, "ClosePort?"=FALSE, "Wait Notifier"=refnum, "wait for reply"=FALSE} ("Close Port Argument"), Variant=w293) -> (data=w291:T8, error out=w294:errorcluster)
            n123 = Unbundle By Name(w291) -> ("Wait Notifier"=w290:refnum<notifier>, "wait for reply"=w289:bool)  [unwired: 2 out]
            n124 = call-dynamic "Close Port.vi"("Serial Base in"=w285) -> ("error out"=w280:errorcluster, "Serial Base out"=w283:refnum<class "Serial Base.lvclass">)  [unwired: 9 in]
            n125 = Bundle By Name(cluster=T17 {"error"={"status"=FALSE, "code"=0, "source"=""}} ("Close Port (Reply Payload)"), "error"=w280) -> (w288:T17)
            n126 = case shown="True" w289 {
              tunnel: w290 -> [_ w297]
              tunnel: w288 -> [_ w296]
              frame False {
              }
              frame True {
                n127 = Send Notification(notification=w296, notifier=w297) -> ()  [unwired: 1 in, 2 out]
              }
            }
            n128 = Bundle By Name(cluster=w284, "Serial Com Obj"=w283) -> (w282:T2)
            n129 = call "Port Did Close.vi"("Reply Payload"=w288) -> ("error out"=w281:errorcluster)  [unwired: 10 in]
            n130 = Merge Errors(w281, w280, w294) -> (w286:errorcluster)
          }
          frame "Read Buffer" {
            # "It will read the data in the serial port buffer"
            n131 = Unbundle By Name(w302) -> ("Serial Com Obj"=w306:refnum<class "Serial Base.lvclass">)
            n132 = Variant To Data(error in=w316, type=T9 {"Module ID"=-1, "pre-read delay"=-1, "Wait Notifier"=refnum, "wait for reply"=FALSE} ("Read Buffer Argument"), Variant=w314) -> (data=w312:T9, error out=w315:errorcluster)
            n133 = Unbundle By Name(w312) -> ("pre-read delay"=w305:i16, "Wait Notifier"=w311:refnum<notifier>, "wait for reply"=w310:bool)  [unwired: 1 out]
            n134 = call-dynamic "Read buffer.vi"("pre-read delay"=w305, "Serial Base in"=w306) -> ("error out"=w298:errorcluster, "return count"=w304:u32, "buffer output"=w303:string, "Serial Base out"=w301:refnum<class "Serial Base.lvclass">)  [unwired: 6 in]
            n135 = Bundle By Name(cluster=T18 {"buffer output"="", "bytes count"=0, "error"={"status"=FALSE, "code"=0, "source"=""}} ("Read Buffer (Reply Payload)"), "buffer output"=w303, "bytes count"=w304, "error"=w298) -> (w309:T18)
            n136 = case shown="True" w310 {
              tunnel: w311 -> [_ w318]
              tunnel: w309 -> [_ w317]
              frame False {
              }
              frame True {
                n137 = Send Notification(notification=w317, notifier=w318) -> ()  [unwired: 1 in, 2 out]
              }
            }
            n138 = Bundle By Name(cluster=w302, "Serial Com Obj"=w301) -> (w300:T2)
            n139 = call "Read Buffer broadcast.vi"("Reply Payload"=w309) -> ("error out"=w299:errorcluster)  [unwired: 10 in]
            n140 = Merge Errors(w299, w298, w315) -> (w307:errorcluster)
          }
          frame "Send" {
            # "It will send data into the serial port buffer"
            n141 = Unbundle By Name(w323) -> ("Serial Com Obj"=w326:refnum<class "Serial Base.lvclass">)
            n142 = Variant To Data(error in=w336, type=T10 {"Module ID"=-1, "data"="", "Wait Notifier"=refnum, "wait for reply"=FALSE} ("Send Argument"), Variant=w334) -> (data=w332:T10, error out=w335:errorcluster)
            n143 = Unbundle By Name(w332) -> ("data"=w324:string, "Wait Notifier"=w331:refnum<notifier>, "wait for reply"=w330:bool)  [unwired: 1 out]
            n144 = call-dynamic "Send.vi"("data"=w324, "Serial Base in"=w326) -> ("error out"=w319:errorcluster, "bytes count"=w325:u32, "Serial Base out"=w321:refnum<class "Serial Base.lvclass">)  [unwired: 7 in]
            n145 = Bundle By Name(cluster=w323, "Serial Com Obj"=w321) -> (w322:T2)
            n146 = Bundle By Name(cluster=T19 {"bytes count sent"=0, "error"={"status"=FALSE, "code"=0, "source"=""}} ("Send (Reply Payload)"), "bytes count sent"=w325, "error"=w319) -> (w329:T19)
            n147 = case shown="True" w330 {
              tunnel: w331 -> [_ w338]
              tunnel: w329 -> [_ w337]
              frame False {
              }
              frame True {
                n148 = Send Notification(notification=w337, notifier=w338) -> ()  [unwired: 1 in, 2 out]
              }
            }
            n149 = call "Send Broadcast.vi"("Reply Payload"=w329) -> ("error out"=w320:errorcluster)  [unwired: 10 in]
            n150 = Merge Errors(w320, w319, w335) -> (w327:errorcluster)
          }
          frame "Send Line" {
            # "It will send data with the selected termination character to the serial port buffer"
            n151 = Unbundle By Name(w345) -> ("Serial Com Obj"=w344:refnum<class "Serial Base.lvclass">)
            n152 = Variant To Data(error in=w355, type=T11 {"Module ID"=-1, "Termination Char"=enum."none", "data"="", "Wait Notifier"=refnum, "wait for reply"=FALSE} ("Send Line Argument"), Variant=w353) -> (data=w351:T11, error out=w354:errorcluster)
            n153 = Unbundle By Name(w351) -> ("Termination Char"=w343:T12, "data"=w342:string, "Wait Notifier"=w350:refnum<notifier>, "wait for reply"=w349:bool)  [unwired: 1 out]
            n154 = call-dynamic "Send Line.vi"("Termination Char"=w343, "data"=w342, "Serial Base in"=w344) -> ("error out"=w339:errorcluster, "bytes count"=w341:u32)  [unwired: 6 in, 1 out]
            n155 = Bundle By Name(cluster=T20 {"bytes count"=0, "error"={"status"=FALSE, "code"=0, "source"=""}} ("Send Line (Reply Payload)"), "bytes count"=w341, "error"=w339) -> (w348:T20)
            n156 = case shown="True" w349 {
              tunnel: w350 -> [_ w357]
              tunnel: w348 -> [_ w356]
              frame False {
              }
              frame True {
                n157 = Send Notification(notification=w356, notifier=w357) -> ()  [unwired: 1 in, 2 out]
              }
            }
            n158 = call "Send Line broadcast.vi"("Reply Payload"=w348) -> ("error out"=w340:errorcluster)  [unwired: 10 in]
            n159 = Merge Errors(w340, w339, w354) -> (w346:errorcluster)
          }
          frame "---Copy This Frame---" {
            # "Duplicate this frame when creating new messages.  Change this comment in the duplicated frame to describe this message."
            n160 = Merge Errors(w360) -> (w359:errorcluster)
          }
          frame "---Exit and Error Handling---" {
            # "Separator - the following cases handle errors and exit messages."
          }
          frame "Error" {
            # "#CodeRecommended - If you ever change the name of this \"Error\" message, you'll need to update the name in the Check Loop Error.vi as well."
            # "#CodeRecommended - If the module is running in standalone mode (External Launch = FALSE), this code will pop up an error dialog and call the 'Exit' message if an error occurs. Add more fine-grained error handling here."
            # "Error - Check the error message data and respond accordingly. This message is sent by the \"Error Handler\" VIs at the end of each loop in this application."
            n161 = property class="Mod Admin"(reference=w366) -> ("Accessors:External Launch"=w365:bool, "Accessors:Module ID"=w363:i32)  [unwired: 1 in, 2 out]
            n162 = Variant To Data(error in=w373, type=errorcluster {"status"=FALSE, "code"=0, "source"=""} ("error constant"), Variant=w367) -> (data=w374:errorcluster, error out=w371:errorcluster)
            n163 = call "Error Reported.vi"("Error"=w374, "Module ID"=w363) -> ()  [unwired: 9 in, 1 out]
            n164 = case shown="False" w365 {
              tunnel: [w379 _] -> w370
              tunnel: w364 -> [w377 _]
              tunnel: w374 -> [w378 _]
              frame False {
                # "If the module is running standalone, then pop up an error dialog and call the \"Exit\" message."
                n165 = call <vilib>:"Simple Error Handler.vi"("error in (no error)"=w378) -> ()  [unwired: 4 in, 5 out]
                n166 = call-poly <vilib>:"Delacor_lib_QMH_Enqueue Message (poly).vi"("Priority Message? (F)"=TRUE, "Message"="Exit", "Message Queue in"=w377) -> ("error out"=w379:errorcluster)  [unwired: 7 in, 1 out]
              }
              frame True {
                # "If the module was launched externally, calling the Error Reported broadcast VI is the only action performed by the \"Error\" message. The module's caller can then process the error appropriately."
              }
            }
            n167 = Merge Errors(w371, w370) -> (w369:errorcluster)
            n168 = local write "error out"(w369) -> ()
          }
          frame "Simulate MHL Error" {
            # "#DQMH_HowTo The 'Simulate MHL Error' button  illustrates how the MHL handles errors. This event is instructional in nature and can be removed."
            # "Simulate an error occurring at the MHL"
            n169 = property class="Mod Admin"(reference=w381) -> ("Accessors:Module ID"=w382:i32)  [unwired: 1 in, 2 out]
            n170 = call "Module Name--constant.vi"("Module ID"=w382) -> ("Module Name"=w380:string)  [unwired: 10 in]
            n171 = xnode "Error Ring"("parameter 0"=w380) -> ("error out"=w384:errorcluster)
            n172 = Merge Errors(w386, w384) -> (w385:errorcluster)
          }
          frame "Exit" {
            w400 = 91  # 91: not all Exit messages will have an argument
            w401 = TRUE  # Stop the VI
            # "Release the message queue reference"
            # "#CodeNeeded - Add any required cleanup code here."
            # "Exit - Exit the application."
            n173 = Variant To Data(error in=w409, type=T4 {"Module ID"=-1, "Origin"="", "Exit via Stop Module Req?"=FALSE, "Wait for Module to stop?"=FALSE} ("Stop Argument"), Variant=w399) -> (data=w396:T4, error out=w404:errorcluster)
            n174 = call <vilib>:"Clear Errors.vi"("error in (no error)"=w404, "specific error code to clear (0: all)"=w400) -> ("error out"=w408:errorcluster)  [unwired: 4 in, 1 out]
            n175 = control-ref of="This VI"() -> (w394:refnum<vi>)
            n176 = call-dynamic "Delacor_lib_QMH_Release Message Queue.vi"("error in"=w408, "Message Queue"=w403) -> ("error out"=w407:errorcluster)  [unwired: 9 in]
            n177 = call "Handle Exit.vi"("Stop Argument"=w396, "Module Admin in"=w395, "VI reference"=w394) -> ("error out"=w405:errorcluster, "Wait for Stop?"=w397:bool)  [unwired: 7 in]
            n178 = Merge Errors(w407, w405) -> (w406:errorcluster)
          }
          frame Default {
            # "'Default' case only runs if there is a message that isn't defined in any of the other cases.  Output a programming error."
            n179 = property class="Mod Admin"(reference=w411) -> ("Accessors:Module ID"=w410:i32)  [unwired: 1 in, 2 out]
            n180 = call "Module Name--constant.vi"("Module ID"=w410) -> ("Module Name"=w412:string)  [unwired: 10 in]
            n181 = xnode "Error Ring"("parameter 0"=w413, "parameter 1"=w412) -> ("error out"=w417:errorcluster)
            n182 = Merge Errors(w415, w417) -> (w416:errorcluster)
          }
        }
        n183 = call-dynamic "Delacor_lib_QMH_Error Handler - Message Handling Loop.vi"("error in"=w214, "Message Queue in"=w204) -> ("dup error in"=w211:errorcluster)  [unwired: 8 in, 1 out]
      }
    }
    frame Error {
      n184 = call "Synchronize Caller Events.vi"("Module Admin"=w431) -> ("Module Admin out"=w430:refnum<class "Delacor_lib_QMH_Cloneable Module Admin.lvclass">)  [unwired: 9 in, 1 out]
      n185 = property class="Mod Admin"(reference=w430) -> ("Accessors:Module ID"=w429:i32)  [unwired: 1 in, 2 out]
      n186 = call-dynamic "Delacor_lib_QMH_Release Message Queue.vi"("error in"=w428, "Message Queue"=w426) -> ("error out"=w427:errorcluster)  [unwired: 9 in]
      n187 = call "Module Name--constant.vi"("Module ID"=w429) -> ("Module Name"=w434:string)  [unwired: 10 in]
      n188 = Format Into String(format string="An error occurred during initialization. %s is no longer running.", w434) -> (resulting string=w432:string)  [unwired: 2 in, 1 out]
      n189 = call "Error Reported.vi"("Additional Information"=w432, "Error"=w427, "Module ID"=w429) -> ()  [unwired: 8 in, 1 out]
    }
  }
  n190 = Merge Errors(w17, w16) -> (w18:errorcluster)
  n191 = call "Close Module.vi"("error in"=w18, "Wait for stop?"=w2, "Module Admin in"=w4) -> ("error out"=w14:errorcluster, "External Launch"=w1:bool, "Module Admin out"=w3:refnum<class "Delacor_lib_QMH_Cloneable Module Admin.lvclass">)  [unwired: 6 in]
  n192 = Unregister For Events(event registration refnum=w9, error in=w14) -> (error out=w13:errorcluster)
  "error out" <- w13
  n193 = local write "Module Admin"(w3) -> ()
  n194 = case "External Launch?" shown="True" w1 {
    tunnel: w13 -> [_ w436]
    frame False {
    }
    frame True {
      n195 = case shown="No Error" w436 {
        frame No Error {
          n196 = invoke class="VI" method="FP.Close"() -> ()  [unwired: 3 in, 3 out]
        }
        frame Error {
          n197 = invoke class="VI" method="FP.Open"("Activate"=TRUE ("Activate?")) -> ()  [unwired: 4 in, 5 out]
        }
      }
    }
  }
